vi "PtInROI.vi"(7 "Point":cluster{"X":i32, "Y":i32}, 8 "error in (no error)":errorcluster, 11 "ROI Descriptor In":T1 {"Contours"."Type" items=["No Selection", "Point", "Line", "Rectangle", "Oval", "Polygon", "Freehand Region", "Annulus", "Unused2", "Unused3", "Broken Line", "Freehand Line", "Rotated Rectangle"]}) -> (0 "error out":errorcluster, 2 "IsInside":bool)   [LabVIEW 2015]
uses:
  IsInsideROI/Release/IsInsideROI.dll
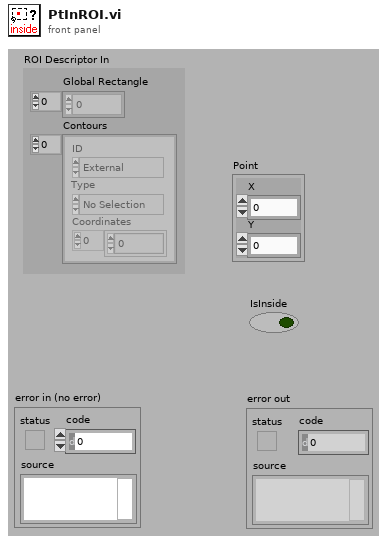
[diagram p1: front panel]
types:
  T1 = typedef "ROI Descriptor" = cluster{"Global Rectangle":i32[], "Contours":cluster{"ID":enum32{"External", "Internal"}, "Type":u32, "Coordinates":i32[]}[]}
  T2 = cluster{"ID":enum32{"External", "Internal"}, "Type":u32, "Coordinates":i32[]}[]
  T3 = cluster{"Global Rectangle[0]":i32, "Global Rectangle[1]":i32, "Global Rectangle[2]":i32, "Global Rectangle[3]":i32}
  T4 = cluster{"Contours[0]":cluster{"ID":enum32{"External", "Internal"}, "Type":u32, "Coordinates":i32[]}}
  T5 = cluster{"ID":enum32{"External", "Internal"}, "Type":u32, "Coordinates":i32[]}
  T6 = cluster{"Coordinates[0]":i32, "Coordinates[1]":i32, "Coordinates[2]":i32, "Coordinates[3]":i32}
  T7 = typedef "IMAQ Rectangle" = cluster{"Left":i32, "Top":i32, "Right":i32, "Bottom":i32, "Rotation":dbl}
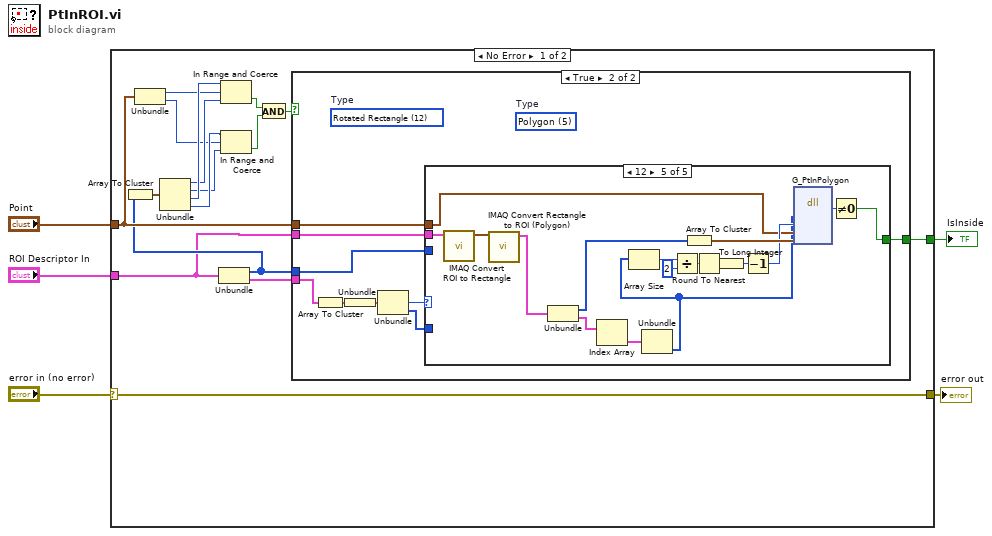
[diagram p0: block diagram]
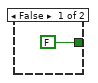
[diagram p2: hidden frame]
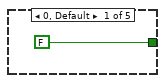
[diagram p3: hidden frame]
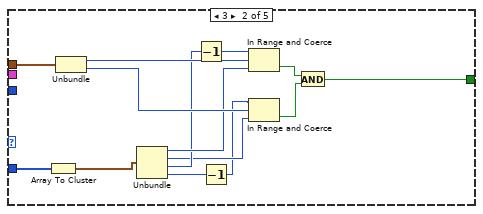
[diagram p4: hidden frame]
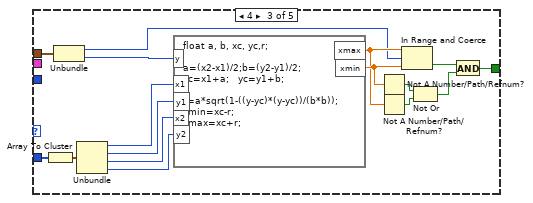
[diagram p5: hidden frame]
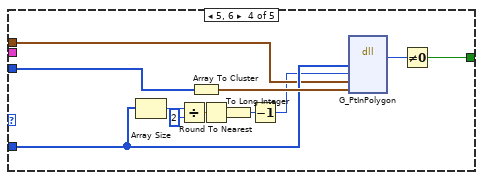
[diagram p6: hidden frame]
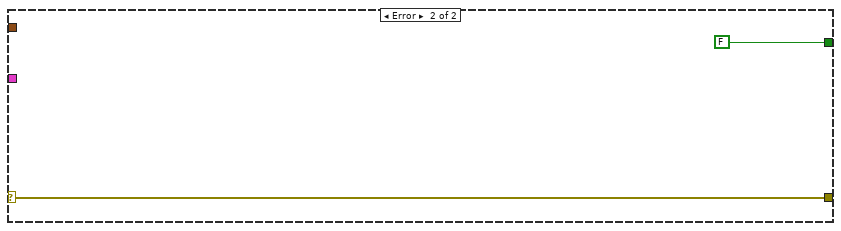
[diagram p7: hidden frame]
diagram:
  n1 = case shown="No Error" "error in (no error)" {
    selector: "error in (no error)" -> [w6 w92]
    tunnel: [w21 FALSE] -> w5
    tunnel: "Point" -> [w10 _]
    tunnel: "ROI Descriptor In" -> [w7 _]
    tunnel: [w6 w92] -> w3
    frame No Error {
      n2 = Unbundle(w10) -> ("X"=w11:i32, "Y"=w12:i32)
      n3 = Unbundle(w7) -> ("Global Rectangle"=w9:i32[], "Contours"=w20:T2)
      n4 = Array To Cluster(array=w9) -> (cluster=w13:T3)
      n5 = Unbundle(w13) -> ("Global Rectangle[0]"=w14:i32, "Global Rectangle[1]"=w15:i32, "Global Rectangle[2]"=w18:i32, "Global Rectangle[3]"=w19:i32)
      n6 = In Range and Coerce(upper limit=w18, x=w11, lower limit=w14) -> (In Range?=w16:bool)  [unwired: 1 out]
      n7 = In Range and Coerce(upper limit=w19, x=w12, lower limit=w15) -> (In Range?=w17:bool)  [unwired: 1 out]
      n8 = And(x=w16, y=w17) -> (x .and. y?=w8:bool)
      n9 = case shown="True" w8 {
        tunnel: [FALSE w30] -> w21
        tunnel: w10 -> [_ w29]
        tunnel: w20 -> [_ w25]
        tunnel: w9 -> [_ w24]
        tunnel: w7 -> [_ w23]
        frame False {
        }
        frame True {
          (unwired) u32 5 items=["No Selection", "Point", "Line", "Rectangle", "Oval", "Polygon", "Freehand Region", "Annulus", "Unused2", "Unused3", "Broken Line", "Freehand Line", "Rotated Rectangle"]  # Type
          (unwired) u32 12 items=["No Selection", "Point", "Line", "Rectangle", "Oval", "Polygon", "Freehand Region", "Annulus", "Unused2", "Unused3", "Broken Line", "Freehand Line", "Rotated Rectangle"]  # Type
          n10 = Array To Cluster(array=w25) -> (cluster=w26:T4)
          n11 = Unbundle(w26) -> ("Contours[0]"=w27:T5)
          n12 = Unbundle(w27) -> ("Type"=w31:u32, "Coordinates"=w28:i32[])  [unwired: 1 out]
          n13 = case shown="12" w31 {
            tunnel: w24 -> [_ _ _ w74 _]
            tunnel: w28 -> [_ w43 w62 w72 _]
            tunnel: w29 -> [_ w46 w60 w71 w81]
            tunnel: [FALSE w35 w48 w64 w75] -> w30
            tunnel: w23 -> [_ _ _ _ w91]
            frame 0, Default {
            }
            frame 3 {
              n14 = Array To Cluster(array=w43) -> (cluster=w42:T6)
              n15 = Unbundle(w46) -> ("X"=w45:i32, "Y"=w44:i32)
              n16 = Unbundle(w42) -> ("Coordinates[0]"=w41:i32, "Coordinates[1]"=w39:i32, "Coordinates[2]"=w40:i32, "Coordinates[3]"=w38:i32)
              n17 = Decrement(x=w40) -> (x-1=w33:i32)
              n18 = Decrement(x=w38) -> (x-1=w34:i32)
              n19 = In Range and Coerce(upper limit=w33, x=w45, lower limit=w41) -> (In Range?=w37:bool)  [unwired: 1 out]
              n20 = In Range and Coerce(upper limit=w34, x=w44, lower limit=w39) -> (In Range?=w36:bool)  [unwired: 1 out]
              n21 = And(x=w37, y=w36) -> (x .and. y?=w35:bool)
            }
            frame 4 {
              n22 = Array To Cluster(array=w62) -> (cluster=w47:T6)
              n23 = Unbundle(w60) -> ("X"=w53:i32, "Y"=w59:i32)
              n24 = Unbundle(w47) -> ("Coordinates[0]"=w61:i32, "Coordinates[1]"=w58:i32, "Coordinates[2]"=w57:i32, "Coordinates[3]"=w56:i32)
              n25 = formula code="float a, b, xc, yc,r;\n\na=(x2-x1)/2;b=(y2-y1)/2;\nxc=x1+a;   yc=y1+b;\n\nr=a*sqrt(1-((y-yc)*(y-yc))/(b*b));\nxmin=xc-r;\nxmax=xc+r;"("x1"=w61, "x2"=w57, "y1"=w58, "y2"=w56, "y"=w59) -> ("xmin"=w55:dbl, "xmax"=w54:dbl)
              n26 = Not A Number/Path/Refnum?(number/path/refnum=w55) -> (NaN/Path/Refnum?=w51:bool)
              n27 = Not A Number/Path/Refnum?(number/path/refnum=w54) -> (NaN/Path/Refnum?=w50:bool)
              n28 = In Range and Coerce(upper limit=w54, x=w53, lower limit=w55) -> (In Range?=w52:bool)  [unwired: 1 out]
              n29 = Not Or(1:w50, 2:w51) -> (0:w49:bool)
              n30 = And(x=w52, y=w49) -> (x .and. y?=w48:bool)
            }
            frame 5, 6 {
              n31 = Array Size(array=w72) -> (size(s)=w70:i32)
              n32 = Divide(x=w70, y=2 ("size(s)")) -> (x/y=w68:dbl)
              n33 = Array To Cluster(array=w74) -> (cluster=w73:T3)
              n34 = Round To Nearest(number=w68) -> (nearest integer value=w67:dbl)
              n35 = To Long Integer(number=w67) -> (32bit integer=w66:i32)
              n36 = Decrement(x=w66) -> (x-1=w65:i32)
              n37 = dll-call lib="J:/Summer Research/SnowDrone/camera/LabVIEW Code/IsInside/IsInsideROI/Release/IsInsideROI.dll" fn="G_PtInPolygon"("Points"=w72, "NPoints"=w65, "ptTest"=w71, "Bounds"=w73) -> ("return type"=w63:i32)  [unwired: 7 in, 2 out]
              n38 = Not Equal To 0?(x=w63) -> (x != 0?=w64:bool)
            }
            frame 12 {
              n39 = call "IMAQ Convert ROI to Rectangle"("ROI Descriptor"=w91) -> ("Rectangle"=w90:T7)  [unwired: 8 in, 1 out]
              n40 = call "IMAQ Convert Rectangle to ROI (Polygon)"("Rectangle"=w90) -> ("ROI Descriptor"=w80:T1)  [unwired: 7 in, 2 out]
              n41 = Unbundle(w80) -> ("Global Rectangle"=w79:i32[], "Contours"=w78:T2)
              n42 = Index Array(array=w78) -> (element=w77:T5)  [unwired: 1 in]
              n43 = Unbundle(w77) -> ("Coordinates"=w76:i32[])  [unwired: 2 out]
              n44 = Array Size(array=w76) -> (size(s)=w88:i32)
              n45 = Divide(x=w88, y=2 ("size(s)")) -> (x/y=w86:dbl)
              n46 = Array To Cluster(array=w79) -> (cluster=w89:T3)
              n47 = Round To Nearest(number=w86) -> (nearest integer value=w85:dbl)
              n48 = To Long Integer(number=w85) -> (32bit integer=w84:i32)
              n49 = Decrement(x=w84) -> (x-1=w83:i32)
              n50 = dll-call lib="J:/Summer Research/SnowDrone/camera/LabVIEW Code/IsInside/IsInsideROI/Release/IsInsideROI.dll" fn="G_PtInPolygon"("Points"=w76, "NPoints"=w83, "ptTest"=w81, "Bounds"=w89) -> ("return type"=w82:i32)  [unwired: 7 in, 2 out]
              n51 = Not Equal To 0?(x=w82) -> (x != 0?=w75:bool)
            }
          }
        }
      }
    }
    frame Error {
    }
  }
  "IsInside" <- w5
  "error out" <- w3
